vi "Pololu.Mgr - Set Device Config.vi"(8 "error in (no error)":errorcluster, 10 "Device Config":T1[](array[typedef]), 11 "PololuCtrl in":refnum<class "PololuCtrl.lvclass">) -> (0 "error out":errorcluster, 3 "PololuCtrl out":refnum<class "PololuCtrl.lvclass">)   [LabVIEW 2018, in "PololuCtrl.lvclass"]
uses:
  PololuCtrl.lvclass
  SubVIs/Pololu.Device Config.ctl
  SubVIs/Pololu.Device Range Config.ctl
  PololuCtrl.lvclass/PololuCtrl.ctl
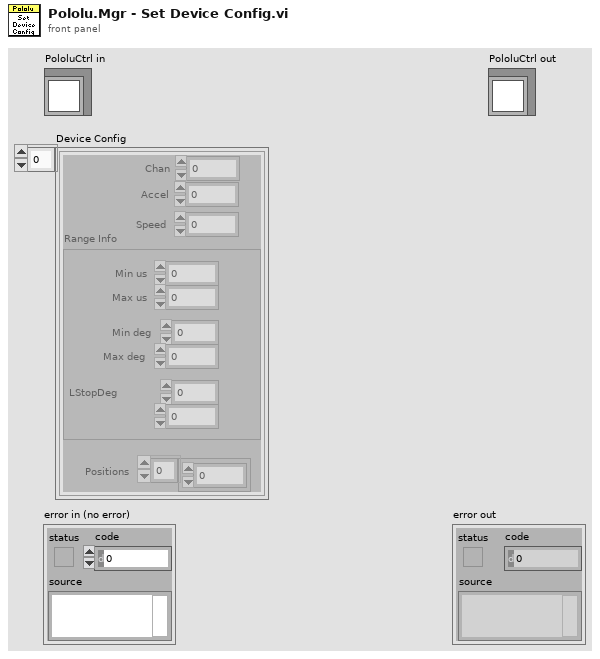
[diagram p1: front panel]
types:
  T1 = typedef "Pololu.Device Config.ctl" = cluster{"Chan":u8, "Accel":u16, "Speed":u16, "Positions":dbl[], "Range Info":T2}
  T2 = typedef "Pololu.Device Range Config.ctl" = cluster{"Min us":dbl, "Max us":dbl, "Min deg":dbl, "Max deg":dbl, "LStopDeg":dbl, "UStopDeg":dbl}
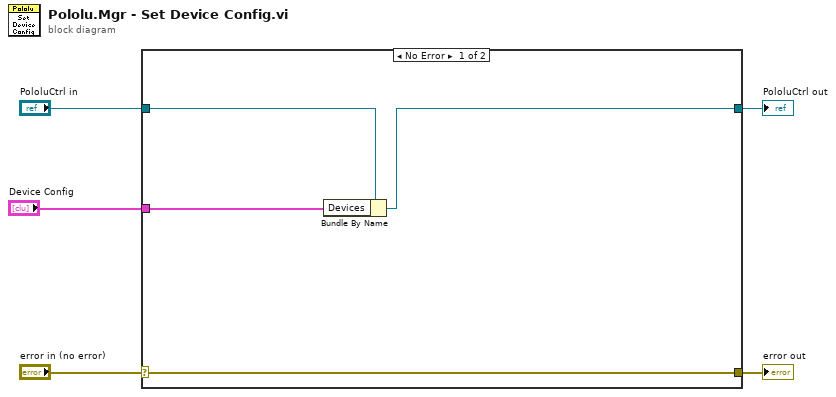
[diagram p0: block diagram]
diagram:
  n1 = case shown="No Error" "error in (no error)" {
    selector: "error in (no error)" -> [w9 w11]
    tunnel: [w9 w11] -> w4
    tunnel: [w8 w10] -> w2
    tunnel: "PololuCtrl in" -> [w7 w10]
    tunnel: "Device Config" -> [w6 _]
    frame No Error {
      n2 = Bundle By Name(cluster=w7, "Devices"=w6) -> (w8:refnum<class "PololuCtrl.lvclass">)
    }
    frame Error {
    }
  }
  "error out" <- w4
  "PololuCtrl out" <- w2
